vi "SetSN (SubVI).vi"(4 "Kinetics Params":path, 6 "UUT":refnum<vi>, 7 "DAQmx Device Name":tag, 9 "Current SN":refnum<vi>, 10 "VISA resource name":refnum<visa-resource-name>, 11 "Next SN":refnum<vi>) -> (0 "error out":errorcluster, 2 "UUT SN Report":string)   [LabVIEW 2017]
uses:
  <vilib>/Utility/config.llb/Write Key (String).vi
  <vilib>/Utility/config.llb/NI_LVConfig.lvlib
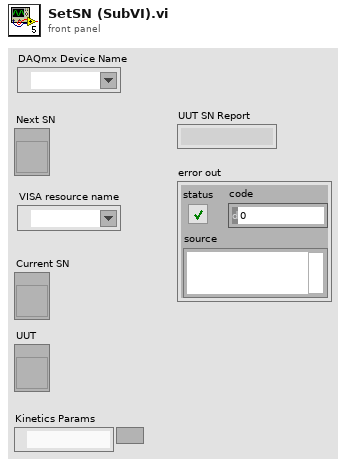
[diagram p1: front panel]
types:
  T1 = enum16{"Init", "0 ohm", "6 ohm", "13.2 ohm", "15 ohm", "25.9 ohm", "33 ohm", "Down", "Up", "Venable", "Firmware", "PowerSuply"}
  T2 = typedef "NI_LVConfig.lvlib/Config Data RefNum.ctl" = refnum<k1>
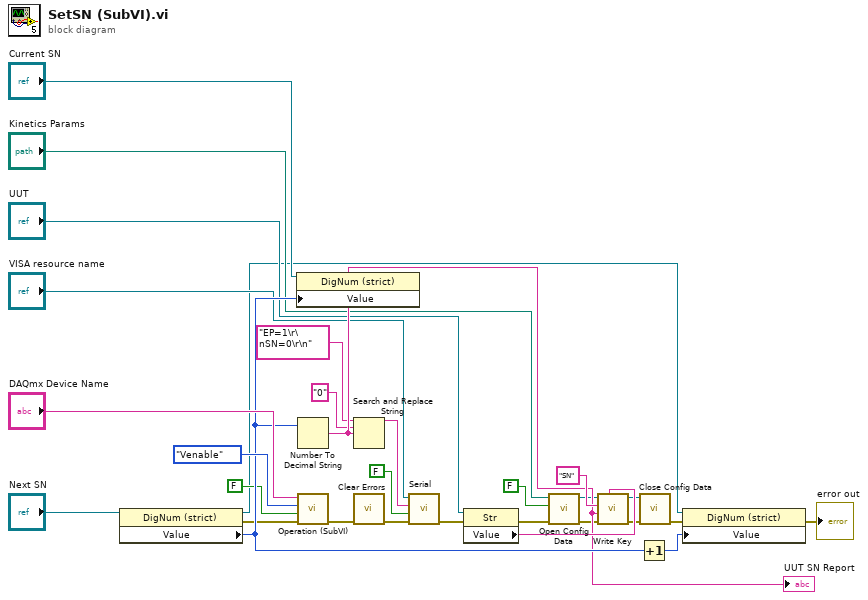
[diagram p0: block diagram]
diagram:
  n1 = property on="Property Node" class="DigNum (strict)"(reference="Next SN") -> (reference out=w5:refnum<vi>, error out=w1:errorcluster, "Value"=w25:i32)  [unwired: 1 in]
  n2 = property on="Property Node" class="DigNum (strict)"(reference="Current SN", "Value"=w25) -> ()  [unwired: 1 in, 2 out]
  n3 = Number To Decimal String(number=w25) -> (decimal integer string=w24:string)  [unwired: 1 in]
  "UUT SN Report" <- w24
  n4 = call "Operation (SubVI).vi"("error in (no error)"=w1, "On/Off"=FALSE, "Operation"=T1."Venable", "DAQmx Device Name"="DAQmx Device Name") -> ("error out"=w23:errorcluster)  [unwired: 7 in]
  n5 = Search and Replace String(input string="EP=1\r\nSN=0\r\n" ("write buffer"), search string="0", replace string=w24) -> (result string=w16:string)  [unwired: 5 in, 3 out]
  n6 = call <vilib>:"Clear Errors.vi"("error in (no error)"=w23) -> ("error out"=w22:errorcluster)  [unwired: 5 in, 1 out]
  n7 = call "Serial.vi"("error in (no error)"=w22, "Clear Log"=FALSE, "write buffer"=w16, "VISA resource name"="VISA resource name") -> ("error out"=w28:errorcluster)  [unwired: 6 in, 1 out]
  n8 = property on="Property Node" class="Str"(reference="UUT", error in=w28) -> (error out=w2:errorcluster, "Value"=w29:string)  [unwired: 1 out]
  n9 = call <vilib>:"Open Config Data.vi"("error in (no error)"=w2, "create file if necessary (T)"=FALSE, "configuration file path"="Kinetics Params") -> ("error out"=w13:errorcluster, "refnum"=w12:T2)  [unwired: 7 out]
  n10 = call-poly <vilib>:"Write Key.vi"("section"=w29, "error in (no error)"=w13, "value"=w24, "key"="SN", "refnum"=w12) -> ("error out"=w19:errorcluster, "refnum out"=w20:T2)  [unwired: 4 in, 1 out]
  n11 = Increment(x=w25) -> (x+1=w6:i32)
  n12 = call <vilib>:"Close Config Data.vi"("error in (no error)"=w19, "refnum"=w20) -> ("error out"=w3:errorcluster)  [unwired: 8 in, 1 out]
  n13 = property on="Property Node" class="DigNum (strict)"(reference=w5, error in=w3, "Value"=w6) -> (error out=→"error out":errorcluster)  [unwired: 1 out]
